vi "DSF.Engine.Memory.Cache.Transfer.Initialize Channels Pointer.vi"(8 "error in (no error)":errorcluster, 10 "Device Ref in":T1=18446744073709551615 format="%.0x", 11 "Transfer Cache in":refnum<class "DSF.Engine.Memory.Cache.Transfer.lvclass">) -> (0 "error out":errorcluster, 3 "Transfer Cache out":refnum<class "DSF.Engine.Memory.Cache.Transfer.lvclass">)   [LabVIEW 2016, in "DSF.Engine.lvlib" / "DSF.Engine.Memory.Cache.Transfer.lvclass"]
uses:
  DSF.Engine.Memory.Cache.Transfer.lvclass
  <vilib>/NI Veristand/Custom Device API/Custom Device Item Ref.ctl
  DSF.Engine.Memory.Cache.Transfer.lvclass/DSF.Engine.Memory.Cache.Transfer.ctl
  Shared/Classes/Transfer/DSF.Shared.Configuration.Transfer.lvclass/DSF.Shared.Configuration.Transfer.ctl
  Shared/VIs/DSF.Shared.Data Type.Sizeof.1D.vi
  Pointer/DSF.Engine.Memory.Pointer.VS Channels.Data Ref to Pointer.vi
  Shared/Classes/Transfer/DSF.Shared.Configuration.Transfer.Get Channel Descriptors.vi
  Shared/Classes/Transfer/DSF.Shared.Configuration.Transfer.Get Direction.vi
  Shared/VIs/DSF.Shared.Data Type.Sizeof.vi
  Pointer/DSF.Engine.Memory.Pointer.VS Channels.lvclass
  C:/Git/SourceTree/DSF/Source/Submodules/Memory/Source/Classes/External/Memory.Pointer.External.lvclass
  Submodules/Memory/Source/Classes/External/Memory.Pointer.External.Encapsulate.vi
  <vilib>/NI Veristand/Custom Device API/Global Data Refs.vi
  <vilib>/NI Veristand/Custom Device API/Custom Device API.lvlib
  Shared/Classes/Transfer/DSF.Shared.Configuration.Transfer.lvclass
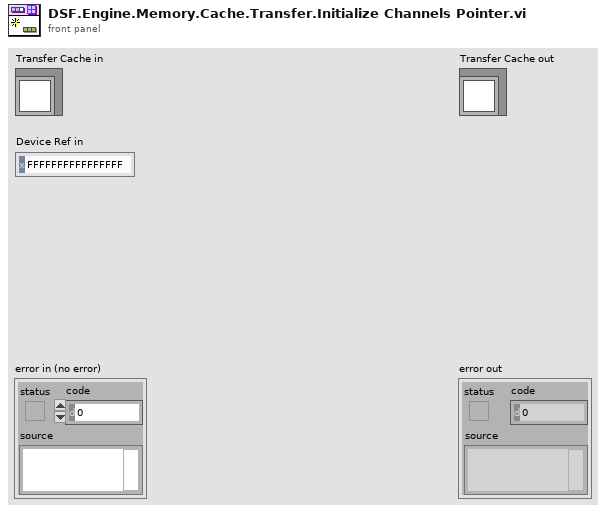
[diagram p1: front panel]
types:
  T1 = typedef "Custom Device API.lvlib/Custom Device Item Ref.ctl" = u64
  T2 = typedef "Custom Device API.lvlib/Data Access Type.ctl" = enum16{"Read", "Write"}
  T3 = typedef "DSF.Shared.lvlib/DSF.Shared.Typedefs.Configuration.Transfer.Channel Block Descriptor.ctl" = cluster{"First Channel Descriptor":T4, "count":u64, "vs channel index":u64}
  T4 = typedef "DSF.Shared.lvlib/DSF.Shared.Typedefs.Configuration.Transfer.Channel Descriptor.ctl" = cluster{"Channel Parameters":T5, "VS Channel Ref":T1}
  T5 = typedef "DSF.Shared.lvlib/DSF.Shared.Typedefs.Configuration.Transfer.Channel Parameters.ctl" = cluster{"offset":u64, "data type":T6}
  T6 = typedef "DSF.Shared.lvlib/DSF.Shared.Typedefs.Data Type.ctl" = enum8{"Bool", "SGL", "DBL", "I8", "I16", "I32", "I64", "U8", "U16", "U32", "U64"}
  T7 = typedef "Custom Device API.lvlib/Data Reference.ctl" = i32
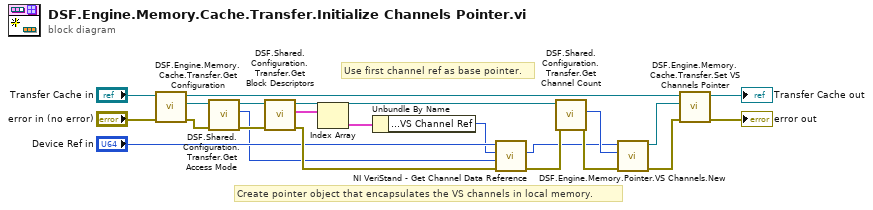
[diagram p0: block diagram]
diagram:
  # "Use first channel ref as base pointer."
  # "Create pointer object that encapsulates the VS channels in local memory."
  n1 = call "DSF.Engine.Memory.Cache.Transfer.Get Configuration.vi"("error in (no error)"="error in (no error)", "Transfer Cache in"="Transfer Cache in") -> ("error out"=w4:errorcluster, "Transfer Configuration"=w6:refnum<class "DSF.Shared.Configuration.Transfer.lvclass">, "Transfer Cache out"=w12:refnum<class "DSF.Engine.Memory.Cache.Transfer.lvclass">)  [unwired: 7 in]
  n2 = call "DSF.Shared.Configuration.Transfer.Get Access Mode.vi"("error in (no error)"=w4, "Transfer Configuration in"=w6) -> ("error out"=w3:errorcluster, "Access"=w2:T2, "Transfer Configuration out"=w5:refnum<class "DSF.Shared.Configuration.Transfer.lvclass">)  [unwired: 7 in]
  n3 = call "DSF.Shared.Configuration.Transfer.Get Block Descriptors.vi"("error in (no error)"=w3, "Transfer Configuration in"=w5) -> ("error out"=w22:errorcluster, "Channel Blocks"=w20:T3[], "Transfer Configuration out"=w11:refnum<class "DSF.Shared.Configuration.Transfer.lvclass">)  [unwired: 7 in]
  n4 = Index Array(array=w20) -> (element=w19:T3)  [unwired: 1 in]
  n5 = Unbundle By Name(w19) -> ("First Channel Descriptor.VS Channel Ref"=w18:T1)
  n6 = call <vilib>:"NI VeriStand - Get Channel Data Reference.vi"("error in (no error)"=w22, "Access"=w2, "Channel Ref in"=w18, "Device Ref in"="Device Ref in") -> ("error out"=w9:errorcluster, "Channel Data Reference"=w7:T7)  [unwired: 5 in, 1 out]
  n7 = call "DSF.Shared.Configuration.Transfer.Get Channel Count.vi"("error in (no error)"=w9, "Transfer Configuration in"=w11) -> ("error out"=w8:errorcluster, "channel count"=w10:u64)  [unwired: 7 in, 1 out]
  n8 = call "DSF.Engine.Memory.Pointer.VS Channels.New.vi"("error in (no error)"=w8, "channel count"=w10, "Data Reference"=w7) -> ("error out"=w16:errorcluster, "VS Channels Pointer out"=w1:refnum<class "DSF.Engine.Memory.Pointer.VS Channels.lvclass">)  [unwired: 7 in]
  n9 = call "DSF.Engine.Memory.Cache.Transfer.Set VS Channels Pointer.vi"("error in (no error)"=w16, "VS Channels Pointer"=w1, "Transfer Cache in"=w12) -> ("error out"=→"error out":errorcluster, "Transfer Cache out"=→"Transfer Cache out":refnum<class "DSF.Engine.Memory.Cache.Transfer.lvclass">)  [unwired: 7 in]
